vi "Preset SERIAL NUMBER.vi"(1 "Serial number":string, 8 "error in (no error)":errorcluster, 11 "VISA resource in":refnum<visa-resource-name>) -> (0 "error out":errorcluster, 3 "VISA resource out":refnum<visa-resource-name>)   [LabVIEW 2025]
uses:
  lot number states--enum.ctl
  <instrlib>/Chroma 19052/Chroma 19052.lvlib
panel:
  # "Min 5 char, Max 13 char"
  # "Set SERIAL number"
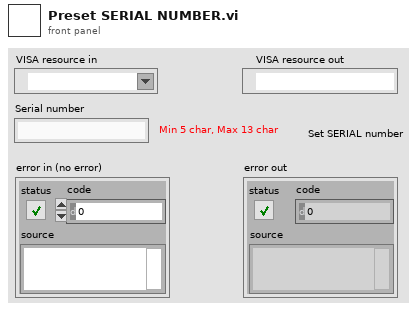
[diagram p1: front panel]
types:
  T1 = typedef "lot number states--enum.ctl" = enum16{"Initialize", "check <=UL", "check >=LL", "Truncate string", "Send command", "Shutdown"}
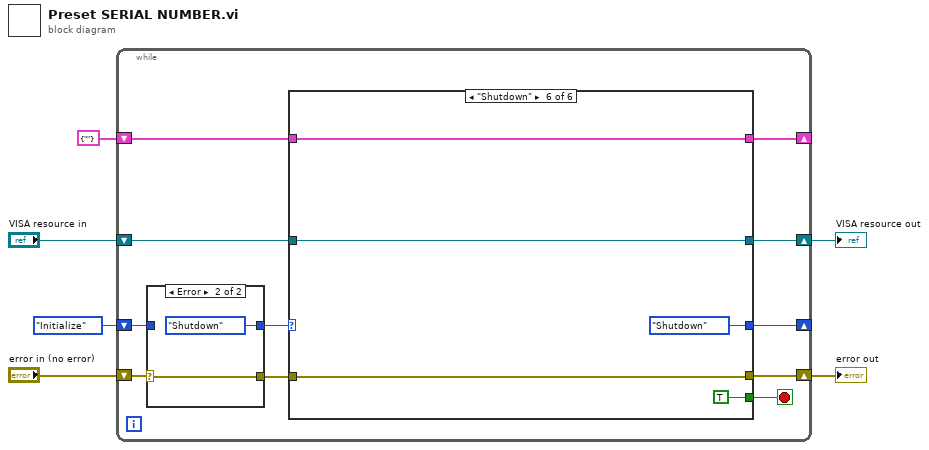
[diagram p0: block diagram]
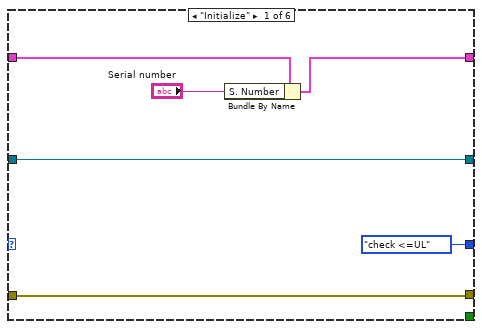
[diagram p3: hidden frame]
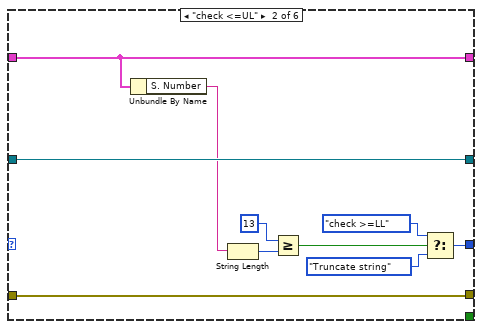
[diagram p4: hidden frame]
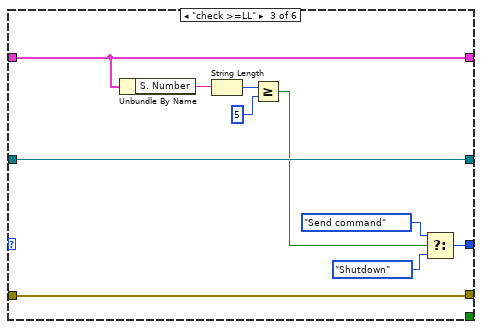
[diagram p5: hidden frame]
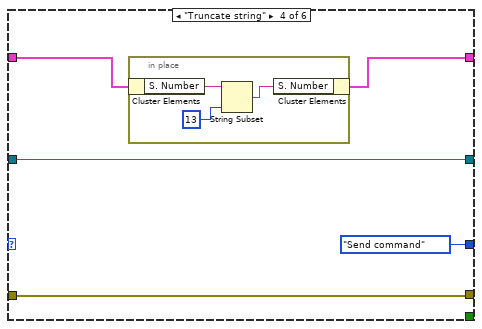
[diagram p6: hidden frame]
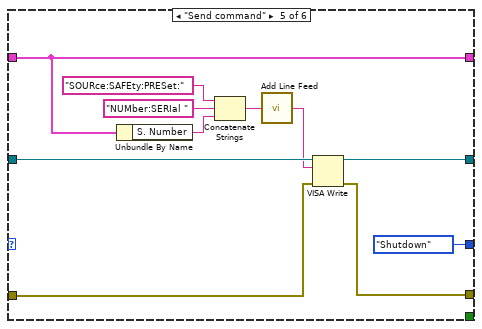
[diagram p7: hidden frame]
diagram:
  n1 = while {
    shift-right: [w14] -> _
    shift-left: lot_number_states--enum."Initialize" -> [w13]
    shift-right: [w8] -> _
    shift-left: cluster{"S. Number":string} {"S. Number"=""} -> [w15]
    shift-right: [w9] -> w3
    shift-left: "VISA resource in" -> [w12]
    shift-right: [w10] -> w4
    shift-left: "error in (no error)" -> [w16]
    stop <- w7 stop-if-true
    n2 = case shown="Error" w16 {
      selector: w16 -> [w19 w20]
      tunnel: [w19 w20] -> w11
      tunnel: [w18 lot_number_states--enum."Shutdown"] -> w17
      tunnel: w13 -> [w18 _]
      frame No Error {
      }
      frame Error {
      }
    }
    n3 = case shown="\"Shutdown\"" w17 {
      tunnel: w15 -> [w24 w29 w39 w49 w59 w69]
      tunnel: [lot_number_states--enum."check <=UL" w34 w43 lot_number_states--enum."Send command" lot_number_states--enum."Shutdown" lot_number_states--enum."Shutdown"] -> w14
      tunnel: w12 -> [w26 w33 w47 w52 w66 w71]
      tunnel: w11 -> [w27 w32 w46 w51 w65 w70]
      tunnel: [w27 w32 w46 w51 w64 w70] -> w10
      tunnel: [w26 w33 w47 w52 w63 w71] -> w9
      tunnel: [w23 w29 w39 w48 w59 w69] -> w8
      tunnel: [_ _ _ _ _ TRUE] -> w7
      frame "Initialize" {
        n4 = Bundle By Name(cluster=w24, "S. Number"="Serial number") -> (w23:cluster{"S. Number":string})
      }
      frame "check <=UL" {
        n5 = Unbundle By Name(w29) -> ("S. Number"=w28:string)
        n6 = String Length(string=w28) -> (length=w36:i32)
        n7 = Greater Or Equal?(x=13 ("y"), y=w36) -> (x >= y?=w35:bool)
        n8 = Select(t=lot_number_states--enum."check >=LL", s=w35, f=lot_number_states--enum."Truncate string") -> (s? t:f=w34:T1)
      }
      frame "check >=LL" {
        n9 = Unbundle By Name(w39) -> ("S. Number"=w38:string)
        n10 = String Length(string=w38) -> (length=w45:i32)
        n11 = Greater Or Equal?(x=w45, y=5) -> (x >= y?=w42:bool)
        n12 = Select(t=lot_number_states--enum."Send command" ("f"), s=w42, f=lot_number_states--enum."Shutdown") -> (s? t:f=w43:T1)
      }
      frame "Truncate string" {
        n13 = in-place {
          n14 = in-place-cluster #1(w49) -> ("S. Number"=w54:string)
          n15 = String Subset(string=w54, length (rest)=13 ("length (rest)")) -> (substring=w53:string)  [unwired: 1 in]
          n16 = in-place-cluster #1("S. Number"=w53) -> (w48:cluster{"S. Number":string})
        }
      }
      frame "Send command" {
        n17 = Unbundle By Name(w59) -> ("S. Number"=w58:string)
        n18 = Concatenate Strings("SOURce:SAFEty:PRESet:", "NUMber:SERIal ", w58) -> (w57:string)
        n19 = call <instrlib>:"Add Line Feed.vi"("Command string"=w57) -> ("Concatenated string"=w56:string)  [unwired: 4 in]
        n20 = VISA Write(VISA resource name=w66, write buffer=w56, error in (no error)=w65) -> (VISA resource name out=w63:refnum<visa-resource-name>, error out=w64:errorcluster)  [unwired: 1 out]
      }
      frame "Shutdown" {
      }
    }
  }
  "error out" <- w4
  "VISA resource out" <- w3
